vi "XIPIN_Video_Processing_Subsystem_1_0.vi"   [LabVIEW 2017]
doc: "Video Processing Subsystem\n------------------------------------\n<b>Need License</b> : Yes"
uses:
  <vilib>/rvi/XilinxIP/XIPIN_XNode/niFpgaXIPIN.xnode
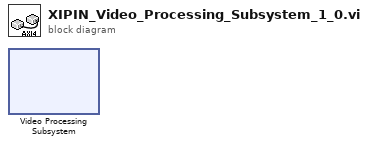
[diagram p0: block diagram]
diagram:
  n1 = xnode ("Video Processing Subsystem")() -> ()
